vi "writefile.vi"(5 "Path":path, 6 "Save&Continue":bool, 7 "Save&Finish":bool, 8 "Polarity":i8, 9 "Sample Rate":i32=1000, 10 "Array":i16[][](array[numeric]), 11 "DescribeWave":T2={"Time"="12:00:00", "Date"="06/09/14", "Specimen"="1", "Location"="EFish Lab", "Species"="Bennetti", "Temp"="25", "Gain"=0, "Coupling"=FALSE, "Comments"="Default values"}) -> (2 "Path Out":path, 3 "Enum":T1)   [LabVIEW 2013]
uses:
  eodrecorderstates.ctl
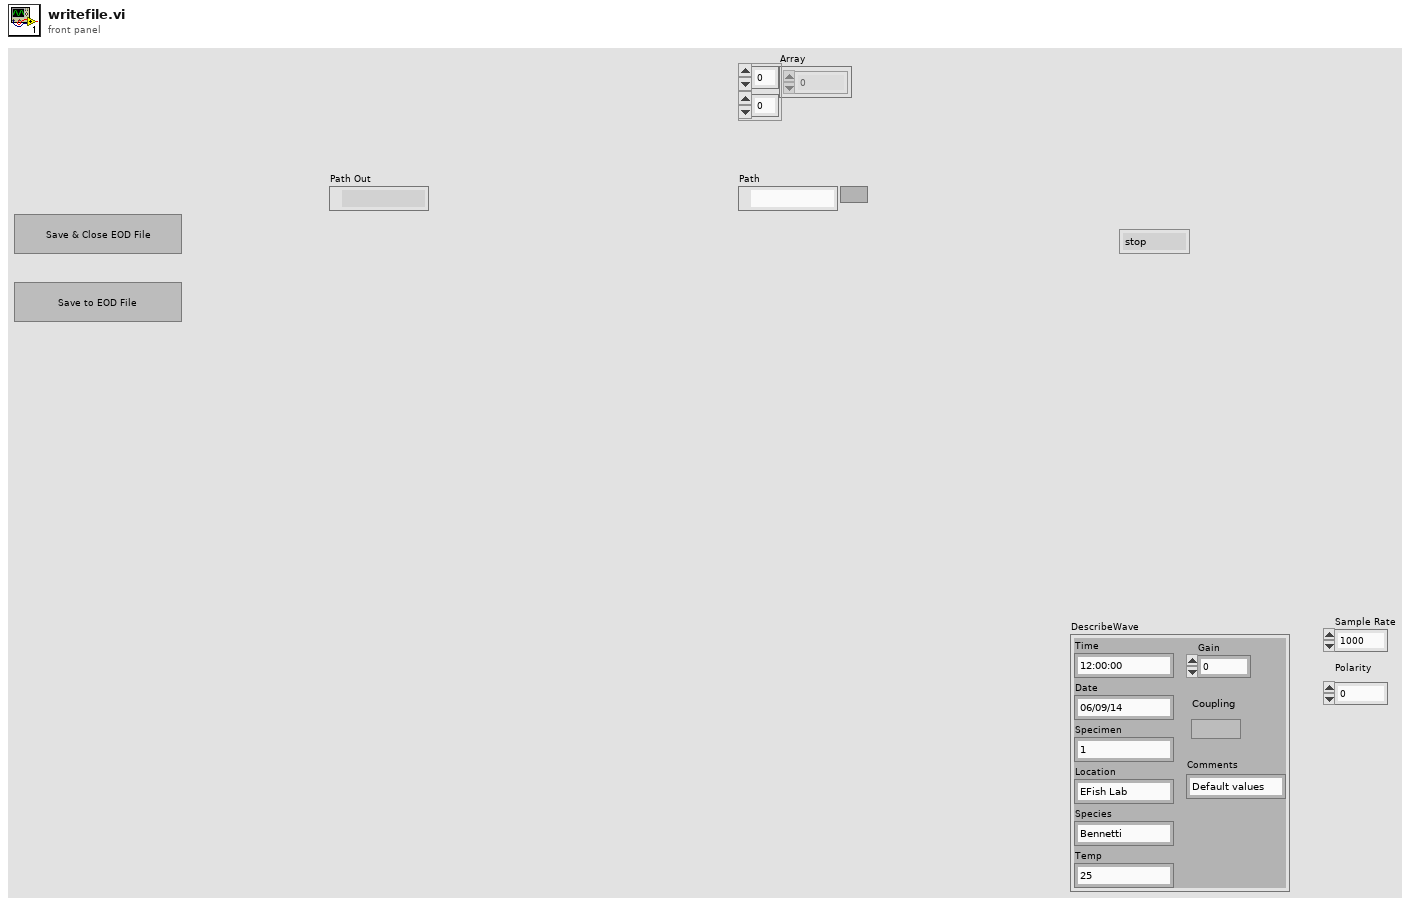
[diagram p1: front panel]
types:
  T1 = typedef "eodrecorderstates.ctl" = enum16{"stop", "initialize", "live data", "capture data", "analyze data", "open data", "display opened data", "write to file"}
  T2 = cluster{"Time":string, "Date":string, "Specimen":string, "Location":string, "Species":string, "Temp":string, "Gain":i32, "Coupling":bool, "Comments":string}
  T3 = enum16{"big-endian, network order", "native, host order", "little-endian"}
  T4 = enum16{"open", "replace", "create", "open or create", "replace or create", "replace or create with confirmation"}
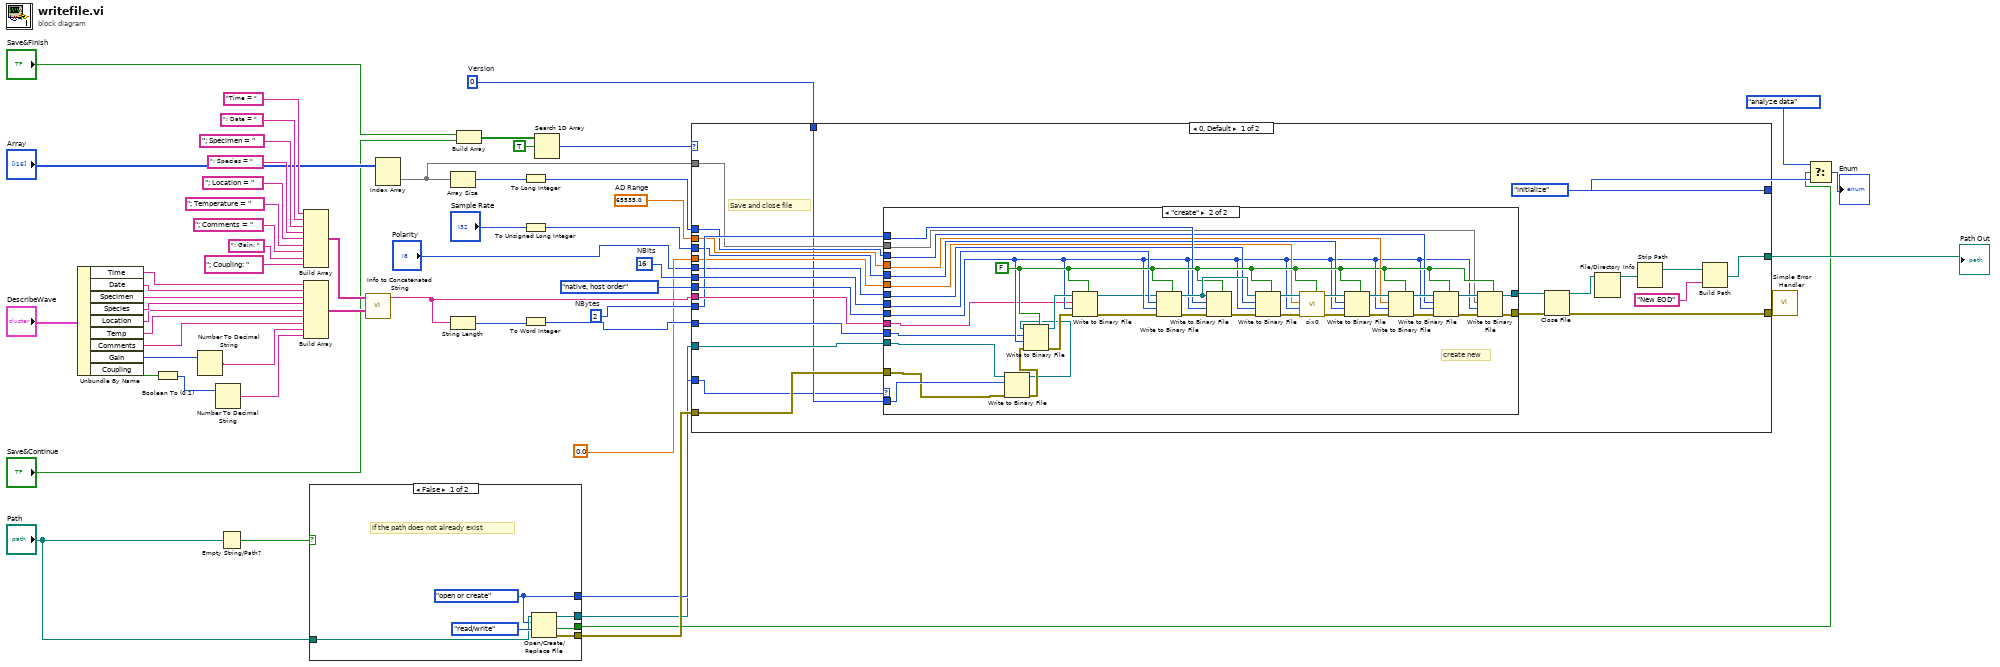
[diagram p0: block diagram]
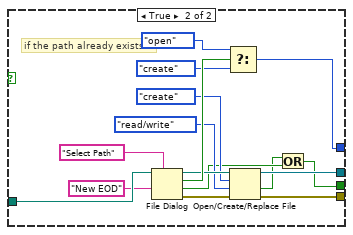
[diagram p2: hidden frame]
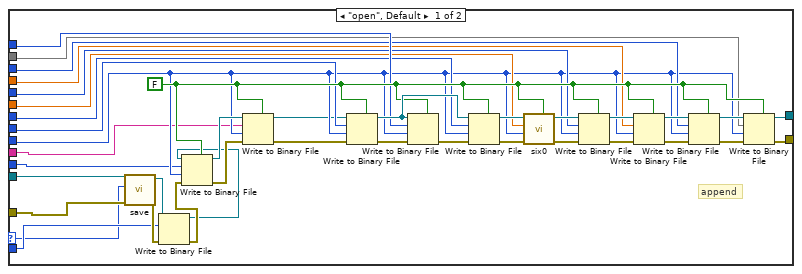
[diagram p3: hidden frame]
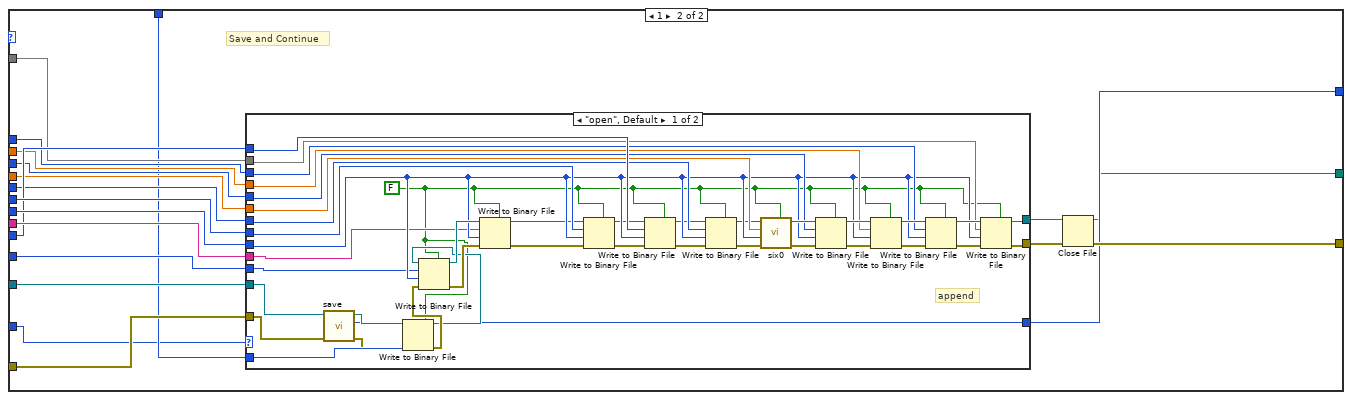
[diagram p4: hidden frame]
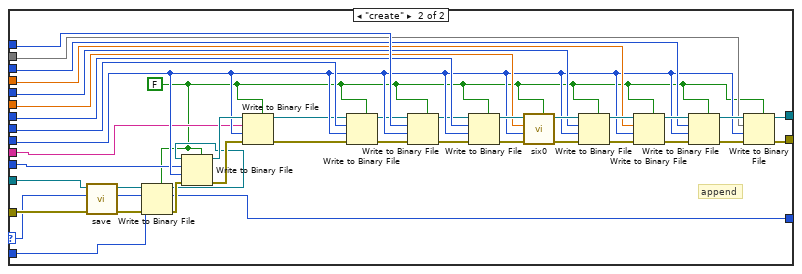
[diagram p5: hidden frame]
diagram:
  w27 = i8 2  # NBytes
  w31 = i8 0  # Version
  w24 = sgl 65535.0  # AD Range
  w28 = i8 16  # NBits
  n1 = Unbundle By Name("DescribeWave") -> ("Time"=w45:string, "Date"=w44:string, "Specimen"=w43:string, "Species"=w42:string, "Location"=w41:string, "Temp"=w40:string, "Comments"=w17:string, "Gain"=w13:i32, "Coupling"=w16:bool)
  n2 = Boolean To (0,1)(Boolean=w16) -> (0, 1=w15:i16)
  n3 = Number To Decimal String(number=w13) -> (decimal integer string=w12:string)  [unwired: 1 in]
  n4 = Number To Decimal String(number=w15) -> (decimal integer string=w14:string)  [unwired: 1 in]
  n5 = Empty String/Path?(string/path="Path") -> (empty?=w6:bool)
  n6 = Build Array("Time = ", "; Date = ", "; Specimen = ", "; Species = ", "; Location = ", "; Temperature = ", "; Comments = ", "; Gain: ", "; Coupling: ") -> (w38:string[])
  n7 = Build Array(w45, w44, w43, w42, w41, w40, w17, w12, w14) -> (w39:string[])
  n8 = case shown="False" w6 {
    tunnel: "Path" -> [w61 w69]
    tunnel: [w60 w72] -> w9
    tunnel: [w59 w71] -> w11
    tunnel: [w58 w74] -> w10
    tunnel: [w57 w64] -> w1
    frame False {
      w58 = T4."open or create" ("operation (0:open)")
      # "if the path does not already exist"
      n9 = Open/Create/Replace File(file path (use dialog)=w61, operation (0:open)=w58, access (0:read/write)=enum16{"read/write", "read-only", "write-only"}."read/write") -> (refnum out=w60:refnum<file>, cancelled=w57:bool, error out=w59:errorcluster)  [unwired: 3 in]
    }
    frame True {
      # "if the path already exists"
      n10 = File Dialog(7:"Select Path", 9:"New EOD", 11:w69) -> (0:w70:errorcluster, 1:w65:bool, 2:w77:bool, 3:w73:path)  [unwired: 4 in]
      n11 = Select(t=T4."open" ("operation (0:open)"), s=w77, f=T4."create" ("operation (0:open)")) -> (s? t:f=w74:T4)
      n12 = Open/Create/Replace File(file path (use dialog)=w73, error in=w70, operation (0:open)=T4."create", access (0:read/write)=enum16{"read/write", "read-only", "write-only"}."read/write") -> (refnum out=w72:refnum<file>, cancelled=w63:bool, error out=w71:errorcluster)  [unwired: 2 in]
      n13 = Or(x=w63, y=w65) -> (x .or. y?=w64:bool)
    }
  }
  n14 = call "Info to Concatenated String.vi"("Info Array"=w39, "Title Array"=w38) -> ("Concatenated\nData"=w29:string)  [unwired: 9 in]
  n15 = Index Array(array="Array") -> (element=w21:i16[])  [unwired: 2 in]
  n16 = Array Size(array=w21) -> (size(s)=w36:i32)
  n17 = String Length(string=w29) -> (length=w37:i32)
  n18 = Build Array("Save&Finish", "Save&Continue") -> (w56:bool[])
  n19 = To Long Integer(number=w36) -> (32bit integer=w23:i32)
  n20 = To Unsigned Long Integer(number="Sample Rate") -> (unsigned 32bit integer=w26:u32)
  n21 = To Word Integer(number=w37) -> (16bit integer=w30:i16)
  n22 = Search 1D Array(1D array=w56, element=TRUE) -> (index of element=w5:i32)  [unwired: 1 in]
  n23 = case shown="0, Default" w5 {
    tunnel: [eodrecorderstates."initialize" w181] -> w4
    tunnel: w11 -> [w101 w197]
    tunnel: w9 -> [w100 w196]
    tunnel: T3."native, host order" ("byte order (0:big-endian, network order)") -> [w99 w195]
    tunnel: [w98 w194] -> w34
    tunnel: w30 -> [w96 w192]
    tunnel: w29 -> [w95 w191]
    tunnel: w28 -> [w94 w190]
    tunnel: w27 -> [w93 w189]
    tunnel: "Polarity" -> [w92 w188]
    tunnel: sgl 0.0 -> [w91 w187]
    tunnel: w26 -> [w90 w186]
    tunnel: w24 -> [w89 w185]
    tunnel: w23 -> [w88 w184]
    tunnel: w21 -> [w87 w183]
    tunnel: w31 -> [w86 w182]
    tunnel: w10 -> [w85 w180]
    tunnel: [w80 w178] -> w8
    frame 0, Default {
      # "Save and close file"
      n24 = case shown="\"create\"" w85 {
        selector: w85 -> [w103 _]
        tunnel: w101 -> [w114 w142]
        tunnel: w100 -> [w104 w143]
        tunnel: w99 -> [w117 w153]
        tunnel: [w112 w149] -> w97
        tunnel: [w113 w150] -> w84
        tunnel: w96 -> [w115 w151]
        tunnel: w95 -> [w116 w152]
        tunnel: w94 -> [w118 w154]
        tunnel: w93 -> [w125 w161]
        tunnel: w92 -> [w119 w155]
        tunnel: w91 -> [w120 w156]
        tunnel: w90 -> [w121 w157]
        tunnel: w89 -> [w122 w158]
        tunnel: w88 -> [w123 w159]
        tunnel: w87 -> [w124 w160]
        tunnel: w86 -> [w109 w147]
        frame "open", Default {
          w126 = FALSE ("prepend array or string size? (T)")
          # "append"
          n25 = call "save.vi"("error in (no error)"=w114, "operation"=w103, "Refnum in"=w104) -> ("error out"=w111:errorcluster, "Refnum out"=w108:refnum<file>)  [unwired: 6 in, 1 out]
          n26 = Write to Binary File(file (use dialog)=w108, data=w109, error in=w111) -> (refnum out=w107:refnum<file>, error out=w110:errorcluster)  [unwired: 3 in, 1 out]
          n27 = Write to Binary File(file (use dialog)=w107, data=w115, error in=w110, 5:w126, 9:w117) -> (refnum out=w141:refnum<file>, error out=w140:errorcluster)  [unwired: 1 in, 1 out]
          n28 = Write to Binary File(file (use dialog)=w141, data=w116, error in=w140, 5:w126, 9:w117) -> (refnum out=w106:refnum<file>, error out=w105:errorcluster)  [unwired: 1 in, 1 out]
          n29 = Write to Binary File(file (use dialog)=w106, data=w118, error in=w105, 5:w126, 9:w117) -> (refnum out=w139:refnum<file>, error out=w138:errorcluster)  [unwired: 1 in, 1 out]
          n30 = Write to Binary File(file (use dialog)=w139, data=w125, error in=w138, 5:w126, 9:w117) -> (error out=w137:errorcluster)  [unwired: 1 in, 2 out]
          n31 = Write to Binary File(file (use dialog)=w139, data=w119, error in=w137, 5:w126, 9:w117) -> (refnum out=w136:refnum<file>, error out=w135:errorcluster)  [unwired: 1 in, 1 out]
          n32 = call "six0.vi"("Boolean"=w126, "error in (no error)"=w135, "byte order (0:big-endian, network order)"=w117, "Numeric"=w120, "Byte Stream File in"=w136) -> ("error out"=w133:errorcluster, "Byte Stream File out"=w134:refnum<file>)  [unwired: 5 in]
          n33 = Write to Binary File(file (use dialog)=w134, data=w121, error in=w133, 5:w126, 9:w117) -> (refnum out=w132:refnum<file>, error out=w131:errorcluster)  [unwired: 1 in, 1 out]
          n34 = Write to Binary File(file (use dialog)=w132, data=w122, error in=w131, 5:w126, 9:w117) -> (refnum out=w130:refnum<file>, error out=w129:errorcluster)  [unwired: 1 in, 1 out]
          n35 = Write to Binary File(file (use dialog)=w130, data=w123, error in=w129, 5:w126, 9:w117) -> (refnum out=w128:refnum<file>, error out=w127:errorcluster)  [unwired: 1 in, 1 out]
          n36 = Write to Binary File(file (use dialog)=w128, data=w124, error in=w127, 5:w126, 9:w117) -> (refnum out=w113:refnum<file>, error out=w112:errorcluster)  [unwired: 1 in, 1 out]
        }
        frame "create" {
          w162 = FALSE ("prepend array or string size? (T)")
          # "create new"
          n37 = Write to Binary File(file (use dialog)=w143, data=w147, error in=w142) -> (refnum out=w146:refnum<file>, error out=w148:errorcluster)  [unwired: 3 in, 1 out]
          n38 = Write to Binary File(file (use dialog)=w146, data=w151, error in=w148, 5:w162, 9:w153) -> (refnum out=w177:refnum<file>, error out=w176:errorcluster)  [unwired: 1 in, 1 out]
          n39 = Write to Binary File(file (use dialog)=w177, data=w152, error in=w176, 5:w162, 9:w153) -> (refnum out=w144:refnum<file>, error out=w145:errorcluster)  [unwired: 1 in, 1 out]
          n40 = Write to Binary File(file (use dialog)=w144, data=w154, error in=w145, 5:w162, 9:w153) -> (refnum out=w175:refnum<file>, error out=w174:errorcluster)  [unwired: 1 in, 1 out]
          n41 = Write to Binary File(file (use dialog)=w175, data=w161, error in=w174, 5:w162, 9:w153) -> (error out=w173:errorcluster)  [unwired: 1 in, 2 out]
          n42 = Write to Binary File(file (use dialog)=w175, data=w155, error in=w173, 5:w162, 9:w153) -> (refnum out=w172:refnum<file>, error out=w171:errorcluster)  [unwired: 1 in, 1 out]
          n43 = call "six0.vi"("Boolean"=w162, "error in (no error)"=w171, "byte order (0:big-endian, network order)"=w153, "Numeric"=w156, "Byte Stream File in"=w172) -> ("error out"=w169:errorcluster, "Byte Stream File out"=w170:refnum<file>)  [unwired: 5 in]
          n44 = Write to Binary File(file (use dialog)=w170, data=w157, error in=w169, 5:w162, 9:w153) -> (refnum out=w168:refnum<file>, error out=w167:errorcluster)  [unwired: 1 in, 1 out]
          n45 = Write to Binary File(file (use dialog)=w168, data=w158, error in=w167, 5:w162, 9:w153) -> (refnum out=w166:refnum<file>, error out=w165:errorcluster)  [unwired: 1 in, 1 out]
          n46 = Write to Binary File(file (use dialog)=w166, data=w159, error in=w165, 5:w162, 9:w153) -> (refnum out=w164:refnum<file>, error out=w163:errorcluster)  [unwired: 1 in, 1 out]
          n47 = Write to Binary File(file (use dialog)=w164, data=w160, error in=w163, 5:w162, 9:w153) -> (refnum out=w150:refnum<file>, error out=w149:errorcluster)  [unwired: 1 in, 1 out]
        }
      }
      n48 = Close File(refnum=w84, error in=w97) -> (path=w82:path, error out=w98:errorcluster)
      n49 = File/Directory Info(path=w82) -> (path out=w83:path)  [unwired: 1 in, 6 out]
      n50 = Strip Path(path=w83) -> (stripped path=w81:path)  [unwired: 1 out]
      n51 = Build Path(base path=w81, name or relative path="New EOD") -> (appended path=w80:path)
    }
    frame 1 {
      # "Save and Continue"
      n52 = case shown="\"open\", Default" w180 {
        selector: w180 -> [_ w238]
        tunnel: w197 -> [w200 w243]
        tunnel: w196 -> [w198 w239]
        tunnel: w195 -> [w216 w256]
        tunnel: [w212 w252] -> w193
        tunnel: [w213 w253] -> w179
        tunnel: w192 -> [w214 w254]
        tunnel: w191 -> [w215 w255]
        tunnel: w190 -> [w217 w257]
        tunnel: w189 -> [w224 w264]
        tunnel: w188 -> [w218 w258]
        tunnel: w187 -> [w219 w259]
        tunnel: w186 -> [w220 w260]
        tunnel: w185 -> [w221 w261]
        tunnel: w184 -> [w222 w262]
        tunnel: w183 -> [w223 w263]
        tunnel: w182 -> [w206 w246]
        tunnel: [w199 w240] -> w181
        frame "open", Default {
          w207 = FALSE ("prepend array or string size? (T)")
          # "append"
          n53 = call "save.vi"("error in (no error)"=w200, "Refnum in"=w198) -> ("error out"=w201:errorcluster, "Recorder State"=w199:T1, "Refnum out"=w202:refnum<file>)  [unwired: 7 in]
          n54 = Write to Binary File(file (use dialog)=w202, data=w206, error in=w201, 5:w207) -> (refnum out=w208:refnum<file>, error out=w209:errorcluster)  [unwired: 2 in, 1 out]
          n55 = Write to Binary File(file (use dialog)=w208, data=w214, error in=w209, 5:w207, 9:w216) -> (refnum out=w237:refnum<file>, error out=w236:errorcluster)  [unwired: 1 in, 1 out]
          n56 = Write to Binary File(file (use dialog)=w237, data=w215, error in=w236, 5:w207, 9:w216) -> (refnum out=w205:refnum<file>, error out=w204:errorcluster)  [unwired: 1 in, 1 out]
          n57 = Write to Binary File(file (use dialog)=w205, data=w217, error in=w204, 5:w207, 9:w216) -> (refnum out=w211:refnum<file>, error out=w235:errorcluster)  [unwired: 1 in, 1 out]
          n58 = Write to Binary File(file (use dialog)=w211, data=w224, error in=w235, 5:w207, 9:w216) -> (refnum out=w210:refnum<file>, error out=w234:errorcluster)  [unwired: 1 in, 1 out]
          n59 = Write to Binary File(file (use dialog)=w210, data=w218, error in=w234, 5:w207, 9:w216) -> (refnum out=w203:refnum<file>, error out=w233:errorcluster)  [unwired: 1 in, 1 out]
          n60 = call "six0.vi"("Boolean"=w207, "error in (no error)"=w233, "byte order (0:big-endian, network order)"=w216, "Numeric"=w219, "Byte Stream File in"=w203) -> ("error out"=w231:errorcluster, "Byte Stream File out"=w232:refnum<file>)  [unwired: 5 in]
          n61 = Write to Binary File(file (use dialog)=w232, data=w220, error in=w231, 5:w207, 9:w216) -> (refnum out=w230:refnum<file>, error out=w229:errorcluster)  [unwired: 1 in, 1 out]
          n62 = Write to Binary File(file (use dialog)=w230, data=w221, error in=w229, 5:w207, 9:w216) -> (refnum out=w228:refnum<file>, error out=w227:errorcluster)  [unwired: 1 in, 1 out]
          n63 = Write to Binary File(file (use dialog)=w228, data=w222, error in=w227, 5:w207, 9:w216) -> (refnum out=w226:refnum<file>, error out=w225:errorcluster)  [unwired: 1 in, 1 out]
          n64 = Write to Binary File(file (use dialog)=w226, data=w223, error in=w225, 5:w207, 9:w216) -> (refnum out=w213:refnum<file>, error out=w212:errorcluster)  [unwired: 1 in, 1 out]
        }
        frame "create" {
          w247 = FALSE ("prepend array or string size? (T)")
          # "append"
          n65 = call "save.vi"("error in (no error)"=w243, "operation"=w238, "Refnum in"=w239) -> ("error out"=w242:errorcluster, "Recorder State"=w240:T1, "Refnum out"=w241:refnum<file>)  [unwired: 6 in]
          n66 = Write to Binary File(file (use dialog)=w241, data=w246, error in=w242, 5:w247) -> (refnum out=w248:refnum<file>, error out=w249:errorcluster)  [unwired: 2 in, 1 out]
          n67 = Write to Binary File(file (use dialog)=w248, data=w254, error in=w249, 5:w247, 9:w256) -> (refnum out=w278:refnum<file>, error out=w277:errorcluster)  [unwired: 1 in, 1 out]
          n68 = Write to Binary File(file (use dialog)=w278, data=w255, error in=w277, 5:w247, 9:w256) -> (refnum out=w245:refnum<file>, error out=w244:errorcluster)  [unwired: 1 in, 1 out]
          n69 = Write to Binary File(file (use dialog)=w245, data=w257, error in=w244, 5:w247, 9:w256) -> (refnum out=w251:refnum<file>, error out=w276:errorcluster)  [unwired: 1 in, 1 out]
          n70 = Write to Binary File(file (use dialog)=w251, data=w264, error in=w276, 5:w247, 9:w256) -> (refnum out=w250:refnum<file>, error out=w275:errorcluster)  [unwired: 1 in, 1 out]
          n71 = Write to Binary File(file (use dialog)=w250, data=w258, error in=w275, 5:w247, 9:w256) -> (refnum out=w274:refnum<file>, error out=w273:errorcluster)  [unwired: 1 in, 1 out]
          n72 = call "six0.vi"("Boolean"=w247, "error in (no error)"=w273, "byte order (0:big-endian, network order)"=w256, "Numeric"=w259, "Byte Stream File in"=w274) -> ("error out"=w271:errorcluster, "Byte Stream File out"=w272:refnum<file>)  [unwired: 5 in]
          n73 = Write to Binary File(file (use dialog)=w272, data=w260, error in=w271, 5:w247, 9:w256) -> (refnum out=w270:refnum<file>, error out=w269:errorcluster)  [unwired: 1 in, 1 out]
          n74 = Write to Binary File(file (use dialog)=w270, data=w261, error in=w269, 5:w247, 9:w256) -> (refnum out=w268:refnum<file>, error out=w267:errorcluster)  [unwired: 1 in, 1 out]
          n75 = Write to Binary File(file (use dialog)=w268, data=w262, error in=w267, 5:w247, 9:w256) -> (refnum out=w266:refnum<file>, error out=w265:errorcluster)  [unwired: 1 in, 1 out]
          n76 = Write to Binary File(file (use dialog)=w266, data=w263, error in=w265, 5:w247, 9:w256) -> (refnum out=w253:refnum<file>, error out=w252:errorcluster)  [unwired: 1 in, 1 out]
        }
      }
      n77 = Close File(refnum=w179, error in=w193) -> (path=w178:path, error out=w194:errorcluster)
    }
  }
  "Path Out" <- w8
  n78 = call <vilib>:"Simple Error Handler.vi"("error in (no error)"=w34) -> ()  [unwired: 4 in, 5 out]
  n79 = Select(t=eodrecorderstates."analyze data" ("Enum"), s=w1, f=w4) -> (s? t:f=→"Enum":T1)
